vi "interface.vi"() -> ()   [LabVIEW 2018]
panel:
  in  "STOP":bool
  in  "START":bool
  # "START & STOP the Robot"
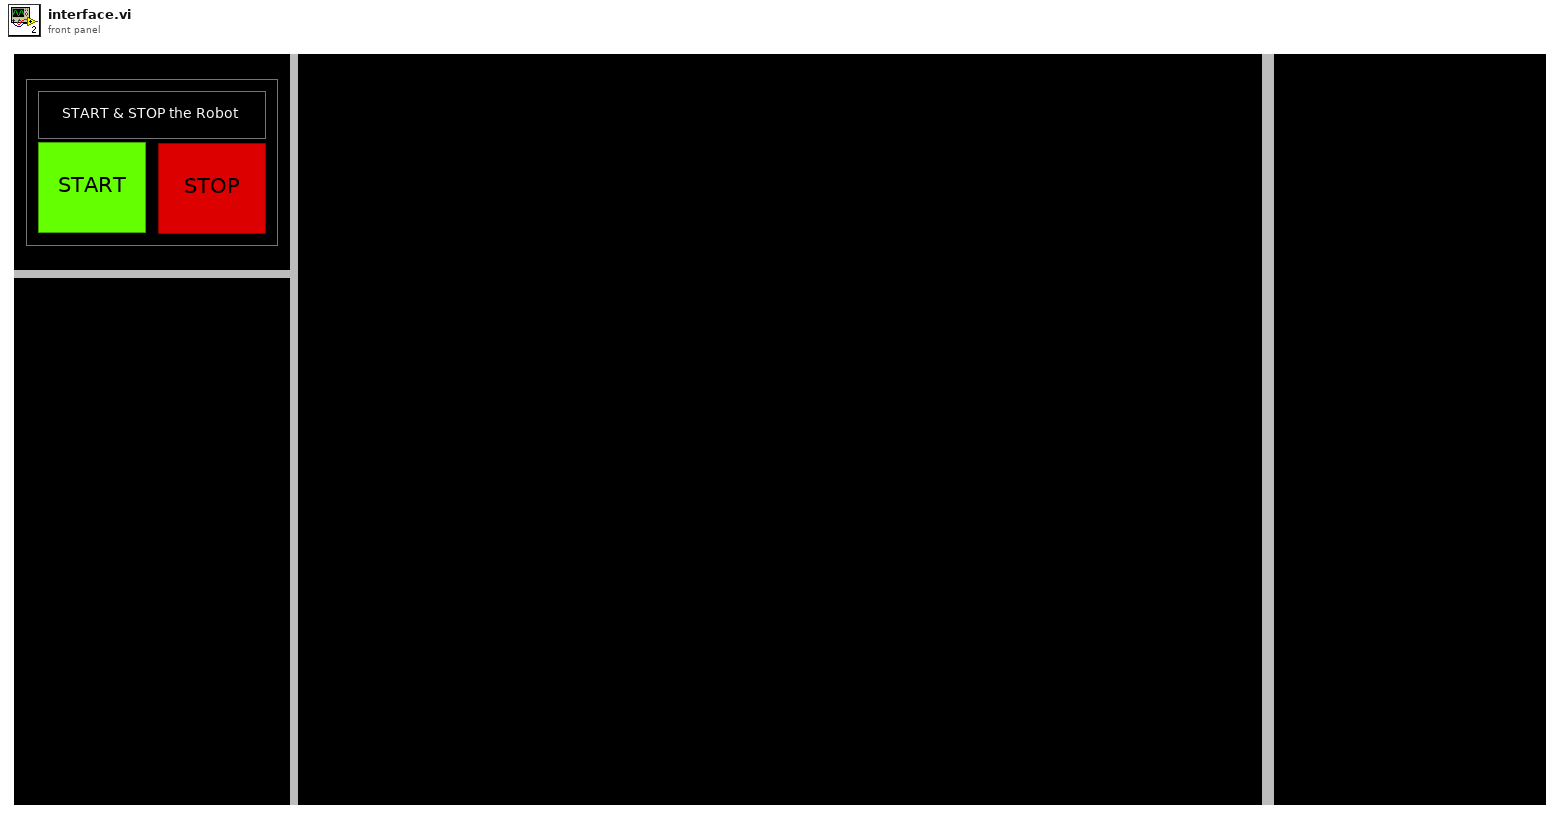
[diagram p1: front panel]
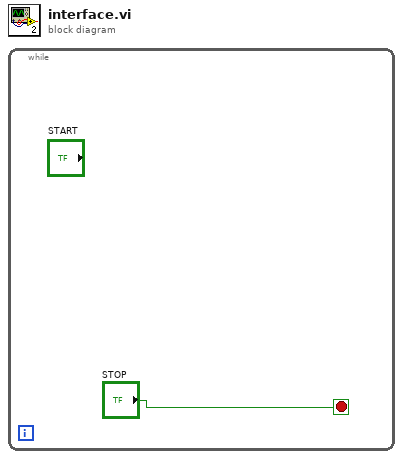
[diagram p0: block diagram]
diagram:
  n1 = while {
    stop <- "STOP" stop-if-true
  }
